vi "subsystem_registerCallbacks_Event.vi"(6 "skipOld":bool, 8 "error in (no error)":errorcluster, 9 "handle":i32, 10 "topic":string="Start", 11 "ProgrammaticInitialization in":refnum<class "ProgrammaticInitialization.lvclass">) -> (0 "error out":errorcluster, 3 "ProgrammaticInitialization out":refnum<class "ProgrammaticInitialization.lvclass">)   [LabVIEW 2016, in "ProgrammaticInitialization.lvclass"]
uses:
  ProgrammaticInitialization.lvclass
  commandType.ctl
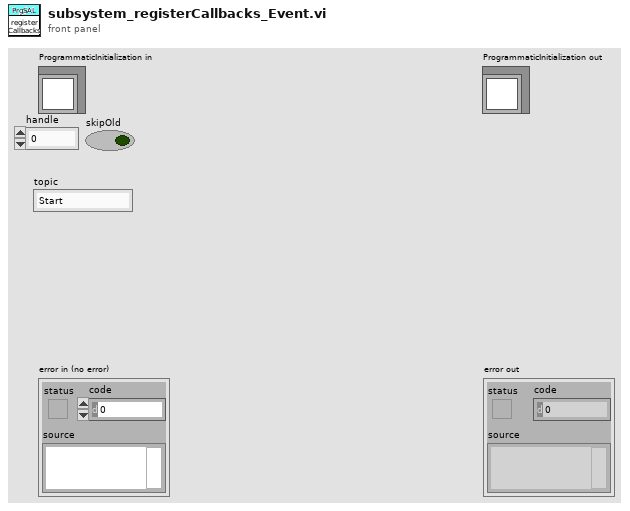
[diagram p1: front panel]
types:
  T1 = typedef "ProgrammaticInitialization.lvclass/commandType.ctl" = enum16{"acceptCommand", "ackCommand", "cancelCallback_command", "cancelCallback_logEvent", "cancelCallback", "flushSamplesEvent", "getEvent", "getNextSample", "getResponse", "getSample", "issueCommand", "logEvent", "monitorCommand", "putSample", "registerCallback_command", "registerCallback_logEvent", "registerCallback", "salCommander", "salEvent", "salProcessor", "salTelemtrySub", "waitForCompletion"}
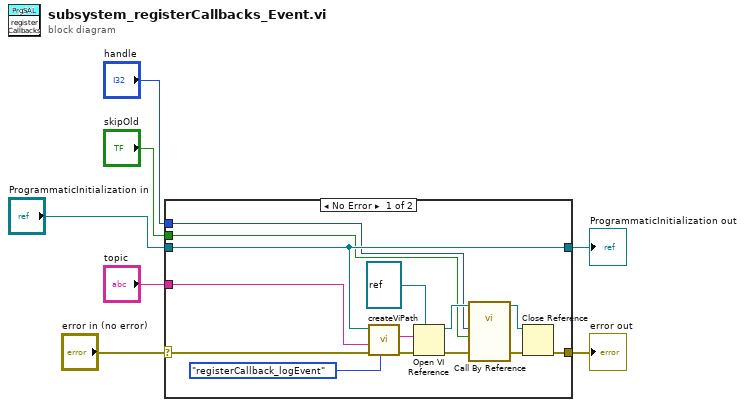
[diagram p0: block diagram]
diagram:
  n1 = case shown="No Error" "error in (no error)" {
    selector: "error in (no error)" -> [w11 w23]
    tunnel: [w10 w23] -> w6
    tunnel: [w12 w22] -> w4
    tunnel: "ProgrammaticInitialization in" -> [w12 w22]
    tunnel: "topic" -> [w13 _]
    tunnel: "handle" -> [w9 _]
    tunnel: "skipOld" -> [w8 _]
    frame No Error {
      n2 = call "createViPath.vi"("CommandType"=commandType."registerCallback_logEvent", "error in (no error)"=w11, "topic"=w13, "ProgrammaticInitialization in"=w12) -> ("error out"=w16:errorcluster, "Vi path"=w15:string)  [unwired: 5 in, 1 out]
      n3 = Open VI Reference(type specifier VI Refnum (for type only)=refnum<vi> refnum, vi path=w15, error in (no error)=w16) -> (vi reference=w17:refnum<vi>, error out=w19:errorcluster)  [unwired: 3 in]
      n4 = call-by-ref "?"(reference=w17, "error in (no error)"=w19, "skipOld"=w8, "handle"=w9) -> (reference out=w18:refnum<vi>, "error out"=w20:errorcluster)  [unwired: 8 in, 2 out]
      n5 = Close Reference(reference=w18, error in (no error)=w20) -> (error out=w10:errorcluster)
    }
    frame Error {
    }
  }
  "error out" <- w6
  "ProgrammaticInitialization out" <- w4
